vi "update全局.vi"() -> ()   [LabVIEW 2016, in "数据传输系统-06.lvlib" / "自动更新.lvlib"]
uses:
  <vilib>/FTP/ftp2.llb/FTP File Info.ctl
  <vilib>/FTP/NI_FTP.lvlib
panel:
  out "path info":T1={"type"=enum."link", "permissions"="", "owner"="", "group"="", "size"=0, "date"="", "name"="", "link name"=""} caption="路径信息"
  in  "updateconfiguration":T2={"主机"="27.154.58.30", "用户"="update", "密码"="std23506", "远程路径"="数据传输系统\\平台数据传输系统.exe", "下载文件名"="平台数据传输系统.exe", "软件版本"=""}
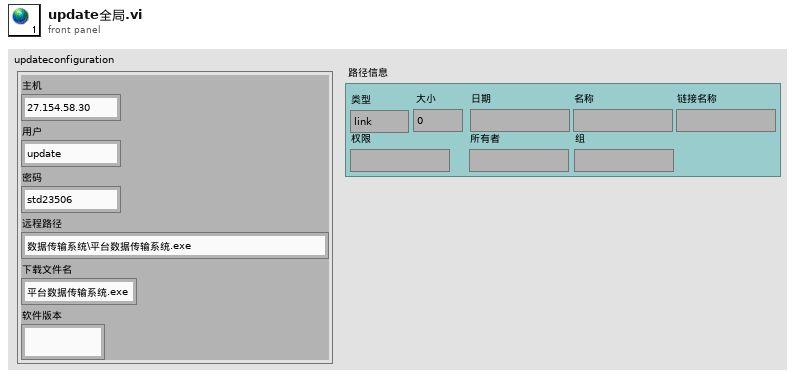
[diagram p1: front panel]
types:
  T1 = typedef "NI_FTP.lvlib/FTP File Info.ctl" = cluster{"type":enum16{"unknown", "file", "dir", "link"}, "permissions":string, "owner":string, "group":string, "size":i32, "date":string, "name":string, "link name":string}
  T2 = cluster{"主机":string, "用户":string, "密码":string, "远程路径":string, "下载文件名":string, "软件版本":string}
diagram:
